vi "svfa_Check Data Valid [FFT subset] (N Ch).vi"(0 "scaled signals":waveform(dbl)[](array[waveform]), 2 "restart averaging (F)":bool, 7 "window":T3=1 items=["None"=0, "Hanning"=1, "Hamming"=2, "Blackman-Harris"=3, "Exact Blackman"=4, "Blackman"=5, "Flat Top"=6, "4 Term B-Harris "=7, "7 Term B-Harris"=8, "Low Sidelobe"=9, "Force"=64, "Exponential"=65, "Blackman Nuttall"=11, "Triangle"=30, "Bartlett-Hanning"=31, "Bohman"=32, "Parzen"=33, "Welch"=34, "Kaiser"=60, "Dolph-Chebyshev"=61, "Gaussian"=62], 9 "averaging parameters":T2={"averaging mode"=enum."No averaging", "weighting mode"=enum."Linear", "number of averages"=10, "linear mode"=enum."Auto restart"}, 11 "error in (no error)":errorcluster, 12 "frequency range in":T1={"start frequency"=20.0, "stop frequency"=20000.0} {"stop frequency" format="%.2f"; "start frequency" format="%.2f"}) -> (3 "restart averaging":bool, 4 "dup scaled signals":waveform(dbl)[](array[waveform]), 8 "window":u16(ring)=1 items=["None "=0, "Hanning"=1, "Hamming"=2, "Blackman-Harris"=3, "Exact Blackman"=4, "Blackman"=5, "Flat Top"=6, "4 Term B-Harris "=7, "7 Term B-Harris"=8, "Low Sidelobe"=9, "Force - Exponential"=10, "Gaussian"=62], 10 "dup averaging parameters":T2={"averaging mode"=enum."No averaging", "weighting mode"=enum."Linear", "number of averages"=10, "linear mode"=enum."Auto restart"}, 14 "frequency range out":T1={"start frequency"=20.0, "stop frequency"=20000.0} {"stop frequency" format="%.2f"; "start frequency" format="%.2f"}, 15 "error out":errorcluster)   [LabVIEW 2017]
uses:
  <vilib>/addons/_NISVFA/_Shared subVIs/Controls/svc_Window.ctl
  <vilib>/addons/_NISVFA/_Shared subVIs/Common/svc_Check for Waveform Parameter Continuity (no state).vi
  <vilib>/addons/_NISVFA/_Shared subVIs/Common/svc_Get SV Channel Info.vi
  <vilib>/addons/_NISVFA/_Shared subVIs/Common/svc_Engineering Units to Unit Label.vi
  <vilib>/addons/_NISVFA/_Shared subVIs/Common/svc_Unit Label to Engineering Units.vi
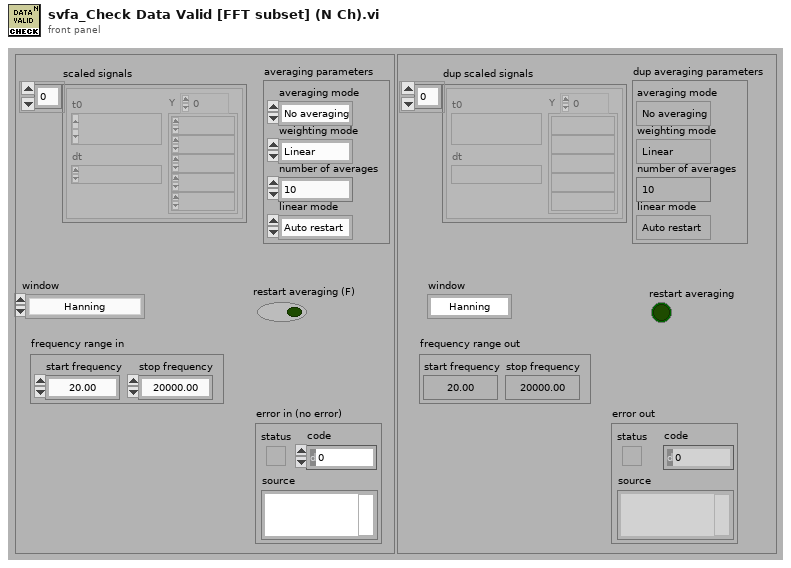
[diagram p1: front panel]
types:
  T1 = cluster{"start frequency":dbl, "stop frequency":dbl}
  T2 = cluster{"averaging mode":enum16{"No averaging", "Vector averaging", "RMS averaging", "Peak hold"}, "weighting mode":enum16{"Linear", "Exponential"}, "number of averages":u32, "linear mode":enum16{"One shot", "Auto restart"}}
  T3 = typedef "svc_Window.ctl" = u32
  T4 = cluster{"dt equal":bool, "array length equal":bool, "number channels change":bool}
  T5 = cluster{"dt":bool, "t0 continuity":bool, "array length":bool, "channel info":bool, "name":bool}
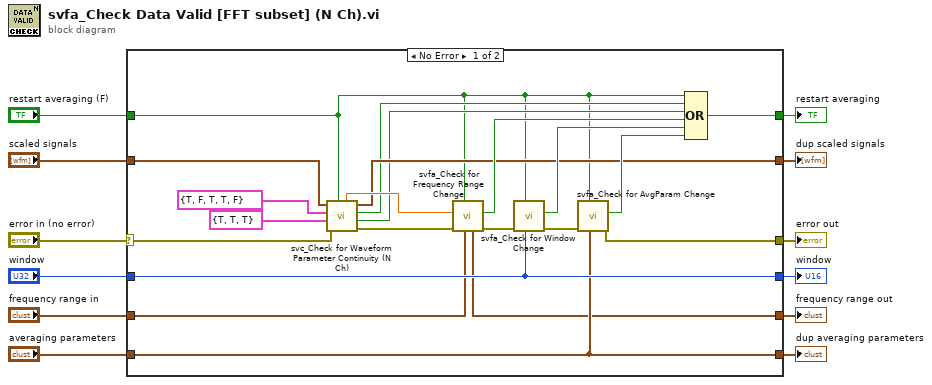
[diagram p0: block diagram]
diagram:
  n1 = case shown="No Error" "error in (no error)" {
    selector: "error in (no error)" -> [w17 w39]
    tunnel: [w15 w39] -> w11
    tunnel: "scaled signals" -> [w22 w37]
    tunnel: "window" -> [w33 w38]
    tunnel: "restart averaging (F)" -> [w16 w34]
    tunnel: [w23 w37] -> w9
    tunnel: [w33 w38] -> w7
    tunnel: "frequency range in" -> [w30 w36]
    tunnel: "averaging parameters" -> [w32 w35]
    tunnel: [w32 w35] -> w4
    tunnel: [w31 w36] -> w3
    tunnel: [w18 w34] -> w1
    frame No Error {
      n2 = call <vilib>:"svc_Check for Waveform Parameter Continuity (N Ch).vi"("restart averaging (F)"=w16, "error in (no error)"=w17, "checks for multichannel parameters"=T4 {"dt equal"=TRUE, "array length equal"=TRUE, "number channels change"=TRUE}, "checks for channel parameter change"=T5 {"dt"=TRUE, "t0 continuity"=FALSE, "array length"=TRUE, "channel info"=TRUE, "name"=FALSE}, "scaled signal(s)"=w22) -> ("error out"=w21:errorcluster, "multichannel parameter changed"=w19:bool, "waveform parameter changed"=w20:bool, "dup scaled signal(s)"=w23:waveform(dbl)[], "dt"=w24:dbl)  [unwired: 2 out]
      n3 = call <vilib>:"svfa_Check for Frequency Range Change.vi"("frequency range in"=w30, "restart averaging (F)"=w16, "error in (no error)"=w21, "dt"=w24) -> ("error out"=w27:errorcluster, "Param_has_changed"=w26:bool, "frequency range out"=w31:T1)  [unwired: 5 in]
      n4 = call <vilib>:"svfa_Check for Window Change.vi"("window"=w33, "restart averaging (F)"=w16, "error in (no error)"=w27) -> ("error out"=w28:errorcluster, "parameter has changed"=w29:bool)  [unwired: 7 in]
      n5 = call <vilib>:"svfa_Check for AvgParam Change.vi"("averaging parameters"=w32, "restart averaging (F)"=w16, "error in (no error)"=w28) -> ("error out"=w15:errorcluster, "parameter has changed"=w25:bool)  [unwired: 7 in]
      n6 = Compound Arithmetic op=OR(w16, w20, w19, w26, w29, w25) -> (w18:bool)
    }
    frame Error {
    }
  }
  "error out" <- w11
  "dup scaled signals" <- w9
  "window" <- w7
  "dup averaging parameters" <- w4
  "frequency range out" <- w3
  "restart averaging" <- w1
